vi "Generate WAMP-SCRAM StoredKey.vi"(9 "Iterations":i32=4096, 10 "Salt":string="3bc3ca01dd1d501ca1c22e1c5d7d16fe", 11 "Secret":string="secret") -> ()   [LabVIEW 2020, in "wamplv.lvlib"]
uses:
  wamplv.lvlib
  Private/Authenticators/WampScramAuthenticator/TypeDefs/HMAC parameters.ctl
  7b673480-243e-4d12-a11e-f93c622d129b.vi
  Private/Authenticators/WampScramAuthenticator/WampScramAuthenticator.lvclass
  Private/Utils/Utils.lvclass
panel:
  out "StoredKey (base64)":string="rSgVdTPamPCbKNnC/LFMJ+A1/RgSi6odgkW6TVz9d8k="
  out "StoredKey (hex)":string="ad28157533da98f09b28d9c2fcb14c27e035fd18128baa1d8245ba4d5cfd77c9"
  in  "Unhashed client key":string="testclientkey"
  # "Note: wamplv only supports PBKDF2 with WAMP-SCRAM. WAMP-SCRAM is experimental and may not work with \nyour router."
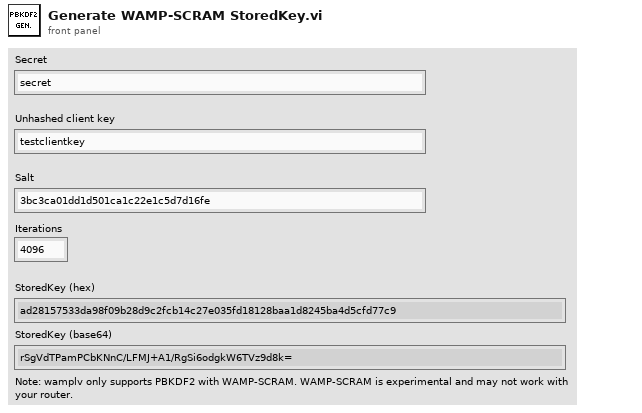
[diagram p1: front panel]
types:
  T1 = typedef "wamplv.lvlib/WampScramAuthenticator.lvclass/HMAC parameters.ctl" = cluster{"Salt":string, "Iterations":i32}
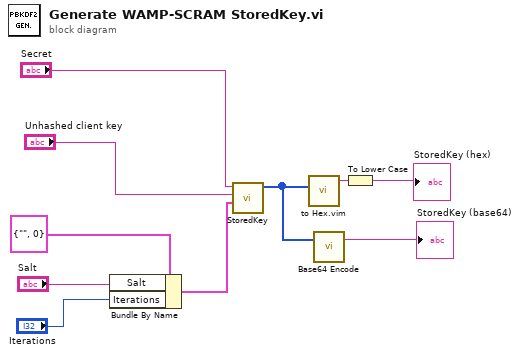
[diagram p0: block diagram]
diagram:
  n1 = Bundle By Name(cluster=T1 {"Salt"="", "Iterations"=0} ("HMAC parameters.ctl"), "Salt"="Salt", "Iterations"="Iterations") -> (w3:T1)
  n2 = call "StoredKey.vi"("HMAC parameters"=w3, "Un-hashed client Key"="Unhashed client key", "Secret"="Secret") -> ("StoredKey"=w2:u8[])  [unwired: 8 in]
  n3 = call "to Hex.vim"("Array"=w2) -> ("Hex string"=w7:string)  [unwired: 2 in]
  n4 = call "Base64 Encode.vi"("Bytes"=w2) -> ("Base64 sring out"=→"StoredKey (base64)":string)  [unwired: 2 in]
  n5 = To Lower Case(string=w7) -> (all lower case string=→"StoredKey (hex)":string)
